vi "Sequence.Read.vi"(8 "error in (no error)":errorcluster, 11 "Recipe file path":path) -> (0 "error out":errorcluster, 2 "Recipe Data":T1[](array[typedef]), 3 "Recipe file path dup":path)   [LabVIEW 2019]
uses:
  typedefs/step.data--Cluster.ctl
  typedefs/step.IO.data--Cluster.ctl
  typedefs/IOType--Enum.ctl
  <vilib>/Utility/file.llb/Read From Spreadsheet File (string).vi
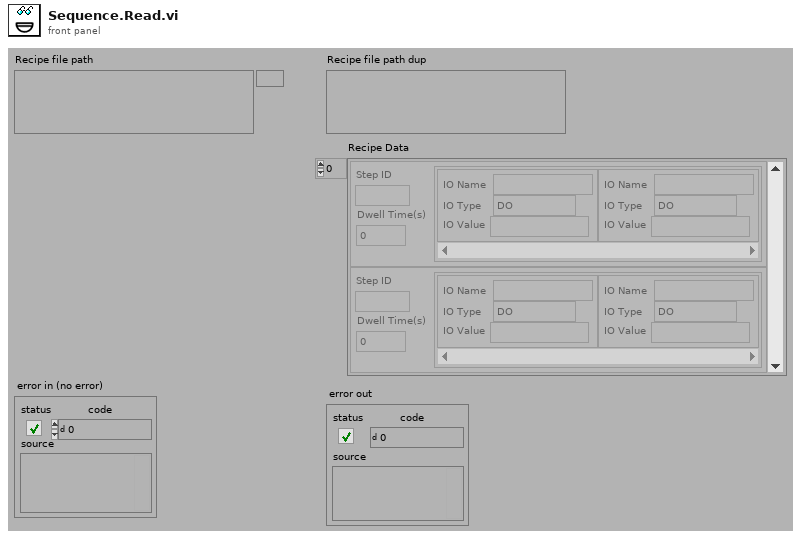
[diagram p1: front panel]
types:
  T1 = typedef "step.data--Cluster.ctl" = cluster{"Step ID":string, "Dwell Time(s)":dbl, "Recipe Step":T2[]}
  T2 = typedef "step.IO.data--Cluster.ctl" = cluster{"IO Name":string, "IO Type":T3, "IO Value":variant}
  T3 = typedef "IOType--Enum.ctl" = enum16{"<Undefined>", "DO", "DI", "AO", "AI"}
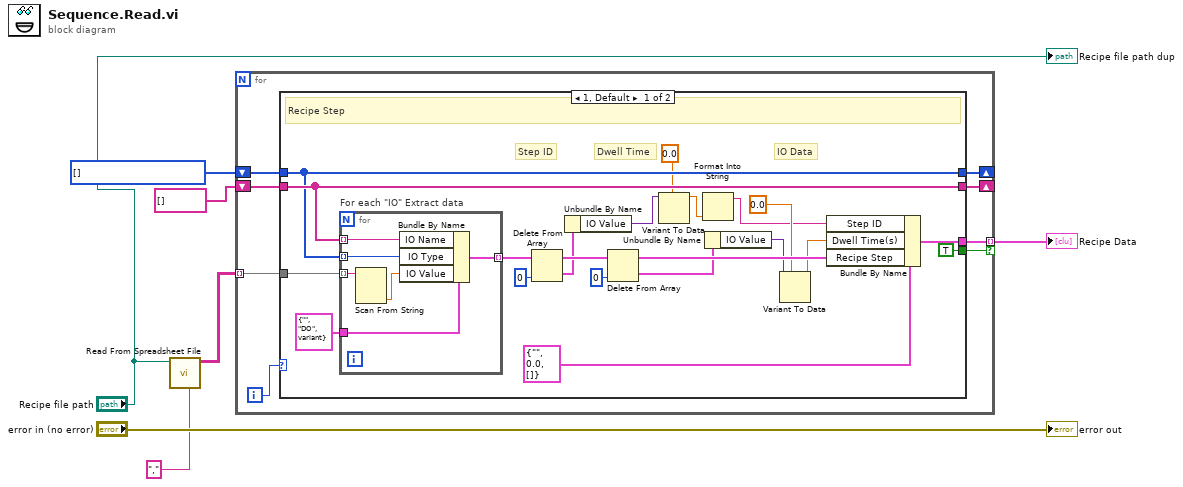
[diagram p0: block diagram]
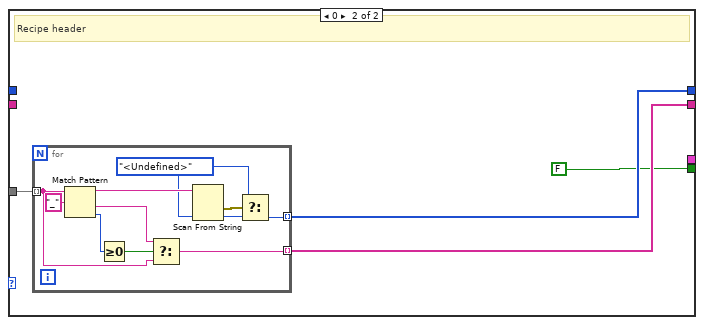
[diagram p2: hidden frame]
diagram:
  w6 = T3[] [] items=["<Undefined>", "DO", "DI", "AO", "AI"]
  n1 = call-poly <vilib>:"Read From Spreadsheet File.vi"("delimiter (\\t)"="," ("delimiter (\\t)"), "file path (dialog if empty)"="Recipe file path") -> ("all rows"=w2:string[][])  [unwired: 5 in, 4 out]
  n2 = for {
    tunnel: w2 -> [w14] mode=indexing
    shift-right: [w13] -> _
    shift-left: w6 -> [w12]
    shift-right: [w11] -> _
    shift-left: string[] [] -> [w10]
    tunnel: [w9] -> w4 mode=indexing if=w8
    i -> [w15]
    n3 = case shown="1, Default" w15 {
      tunnel: w14 -> [w34 w46]
      tunnel: [w35 w45] -> w13
      tunnel: w12 -> [w35 _]
      tunnel: [w36 w44] -> w11
      tunnel: w10 -> [w36 _]
      tunnel: [w21 _] -> w9
      tunnel: [TRUE FALSE] -> w8
      frame 1, Default {
        # "IO Data"
        # "Dwell Time"
        # "Step ID"
        # "Recipe Step"
        n4 = for "For each \"IO\" Extract data" {
          tunnel: w36 -> [w41] mode=indexing
          tunnel: w35 -> [w40] mode=indexing
          tunnel: w34 -> [w39] mode=indexing
          tunnel: T2 {"IO Name"="", "IO Type"=enum."DO", "IO Value"=variant} ("Cluster") -> [w42]
          tunnel: [w37] -> w32 mode=indexing
          n5 = Scan From String(input string=w39) -> (output 1=w38:dbl)  [unwired: 4 in, 3 out]
          n6 = Bundle By Name(cluster=w42, "IO Name"=w41, "IO Type"=w40, "IO Value"=w38) -> (w37:T2)
        }
        n7 = Delete From Array(array=w32, index=0) -> (deleted portion=w26:T2, array with subset deleted=w29:T2[])  [unwired: 1 in]
        n8 = Unbundle By Name(w26) -> ("IO Value"=w19:variant)
        n9 = Delete From Array(array=w29, index=0) -> (deleted portion=w25:T2, array with subset deleted=w27:T2[])  [unwired: 1 in]
        n10 = Variant To Data(type=0.0, Variant=w19) -> (data=w17:dbl)  [unwired: 1 in, 1 out]
        n11 = Format Into String(w17) -> (resulting string=w16:string)  [unwired: 3 in, 1 out]
        n12 = Unbundle By Name(w25) -> ("IO Value"=w24:variant)
        n13 = Variant To Data(type=0.0 ("output 1"), Variant=w24) -> (data=w23:dbl)  [unwired: 1 in, 1 out]
        n14 = Bundle By Name(cluster=T1 {"Step ID"="", "Dwell Time(s)"=0.0, "Recipe Step"=[]} ("Recipe Step"), "Step ID"=w16, "Dwell Time(s)"=w23, "Recipe Step"=w27) -> (w21:T1)
      }
      frame 0 {
        # "Recipe header"
        n15 = for {
          tunnel: w46 -> [w48] mode=indexing
          tunnel: [w52] -> w45 mode=indexing
          tunnel: [w47] -> w44 mode=indexing
          w54 = IOType--Enum."<Undefined>" ("IO Type")
          n16 = Match Pattern(string=w48, regular expression="_") -> (before substring=w56:string, after substring=w49:string, offset past match=w51:i32)  [unwired: 1 in, 1 out]
          n17 = Greater Or Equal To 0?(x=w51) -> (x >= 0?=w50:bool)
          n18 = Select(t=w49, s=w50, f=w48) -> (s? t:f=w47:string)
          n19 = Scan From String(input string=w56, default 1=w54) -> (error out=w55:errorcluster, output 1=w53:T3)  [unwired: 3 in, 2 out]
          n20 = Select(t=w54, s=w55, f=w53) -> (s? t:f=w52:T3)
        }
      }
    }
  }
  "Recipe Data" <- w4
  "Recipe file path dup" <- "Recipe file path"
  "error out" <- "error in (no error)"
